vi "Read Pin.vi"(8 "error in (no error)":errorcluster, 9 "Pin 2":dbl caption="Pin", 10 "Port 4":dbl caption="Port", 11 "Cypress in":refnum<class "Cypress.lvclass">) -> (0 "error out":errorcluster, 3 "Cypress out":refnum<class "Cypress.lvclass">)   [LabVIEW 2020, in "Cypress.lvclass"]
uses:
  Cypress.lvclass
  Cypress.lvclass/Cypress.ctl
  d75e2617-04e3-47b9-aec1-3c41d40c172d.vi
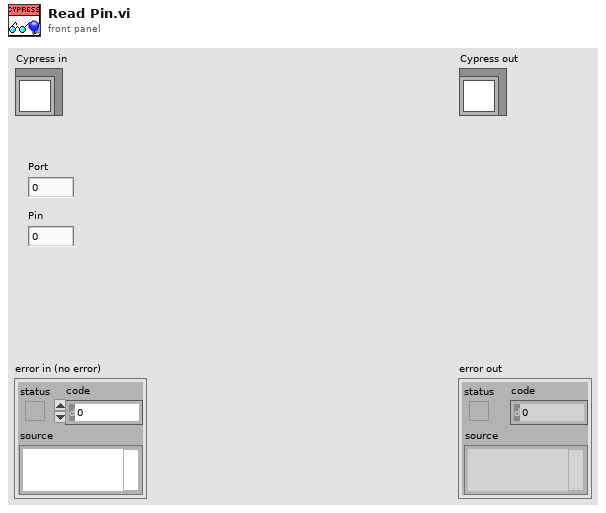
[diagram p1: front panel]
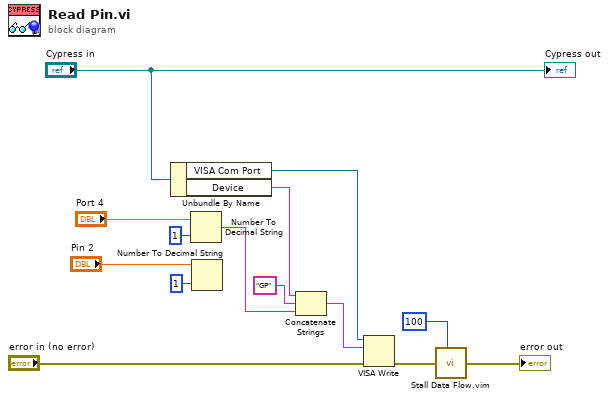
[diagram p0: block diagram]
diagram:
  n1 = Unbundle By Name("Cypress in") -> ("VISA Com Port"=w4:refnum<visa-resource-name>, "Device"=w3:string)
  n2 = Number To Decimal String(number="Port 4", width (-)=i16 1) -> (decimal integer string=w12:string)
  n3 = Number To Decimal String(number="Pin 2", width (-)=i16 1) -> ()  [unwired: 1 out]
  n4 = Concatenate Strings(w3, "GP" ("string"), w12) -> (w13:string)
  n5 = VISA Write(VISA resource name=w4, write buffer=w13, error in (no error)="error in (no error)") -> (error out=w14:errorcluster)  [unwired: 2 out]
  n6 = call "Stall Data Flow.vim"("value in"=w14, "milliseconds to wait"=u32 100) -> ("value out"=→"error out":errorcluster)  [unwired: 1 out]
  "Cypress out" <- "Cypress in"
